vi "Verify.vi"(7 "Actor Layer":refnum<class "Actor Layer.lvclass">, 11 "Actor":T1) -> (2 "Stats":T10, 3 "Actor":T1, 5 "Actor Layer":refnum<class "Actor Layer.lvclass">)   [LabVIEW 2020, in "jettl.lvlib" / "Base.lvlib" / "Actor Layer.lvclass"]
uses:
  Actor Layer.lvclass
  Actor Layer.lvclass/Actor Layer.ctl
  jettl.lvlib
  Msg Set.ctl
  Stats.ctl
  Msg/Msg.lvclass
  Origin.ctl
  Lifecycle.ctl
  Msg Execute Type.ctl
  Msg Attribs.ctl
  Msg.ctl
  Post Setup.ctl
  Pre Setup.ctl
  Actor Attribs.ctl
  Children.ctl
  Actor.ctl
  Layer Type.ctl
  Layer Attribs.ctl
  Layer Map.ctl
  Actor Layer/Actor Layer.lvclass
  Implemented Map.ctl
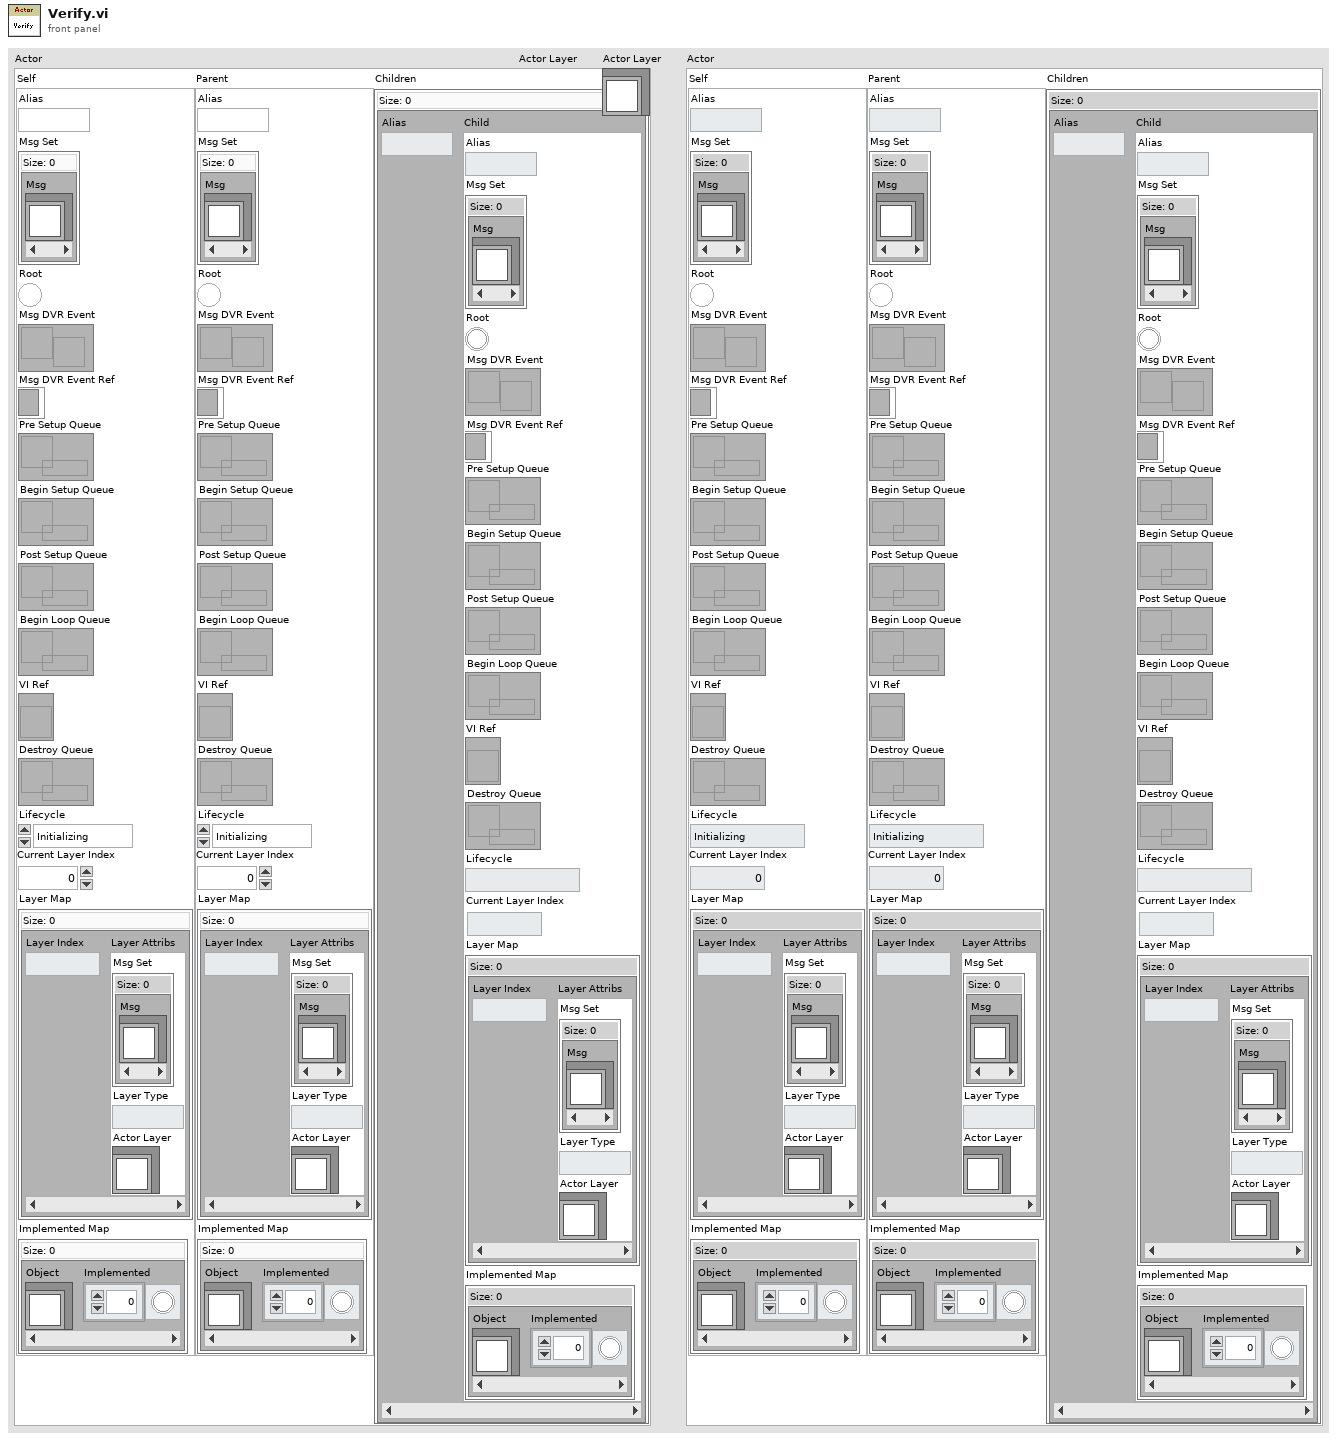
[diagram p1: front panel]
types:
  T1 = typedef "jettl.lvlib/Actor.ctl" = cluster{"Self":T2, "Parent":T2, "Children":T9}
  T2 = typedef "jettl.lvlib/Actor Attribs.ctl" = cluster{"Alias":string, "Msg Set":T3, "Root":bool, "Msg DVR Event":refnum<user-event>, "Msg DVR Event Ref":refnum<event-registration>, "Pre Setup Queue":refnum<queue>, "Begin Setup Queue":refnum<queue>, "Post Setup Queue":refnum<queue>, "Begin Loop Queue":refnum<queue>, "VI Ref":refnum<vi>, "Destroy Queue":refnum<queue>, "Lifecycle":T4, "Current Layer Index":i32, "Layer Map":T5, "Implemented Map":T8}
  T3 = typedef "jettl.lvlib/Msg Set.ctl" = set{refnum<class "Msg.lvclass">}
  T4 = typedef "jettl.lvlib/Lifecycle.ctl" = enum16{"Initializing", "Setting Up", "Starting", "Running", "Stopping", "Tearing Down", "Terminated"}
  T5 = typedef "jettl.lvlib/Layer Map.ctl" = map{i32, T6}
  T6 = typedef "jettl.lvlib/Layer Attribs.ctl" = cluster{"Msg Set":T3, "Layer Type":T7, "Actor Layer":refnum<class "Actor Layer.lvclass">}
  T7 = typedef "jettl.lvlib/Layer Type.ctl" = enum16{"Base", "InnerGlobal", "InnerLocal", "Outer"}
  T8 = typedef "jettl.lvlib/Implemented Map.ctl" = map{refnum<class>, bool[]}
  T9 = typedef "jettl.lvlib/Children.ctl" = map{string, T2}
  T10 = typedef "jettl.lvlib/Stats.ctl" = cluster{"Msg Set":T3}
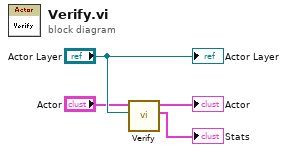
[diagram p0: block diagram]
diagram:
  n1 = call "Verify.vi"("Actor.lvclass"="Actor Layer", "Actor"="Actor") -> ("Stats"=→"Stats":T10, "Actor"=→"Actor":T1)  [unwired: 8 in]
  "Actor Layer" <- "Actor Layer"
